vi "Create Tables.vi"() -> ()   [LabVIEW 2014, in "DB-Configuration.lvlib"]
doc: "This is a utilitiy VI to create necessary configuration tables in Oracle."
uses:
  DB-Configuration.lvlib
  <vilib>/addons/database/Auxilliary.llb/DB Tools Column Info.ctl
  <vilib>/addons/database/Auxilliary.llb/DB Tools DataTypes.ctl
  <vilib>/addons/database/Auxilliary.llb/DB Tools Transaction.ctl
  <vilib>/addons/database/Connection.llb/DB Tools Open Connec (String).vi
  <vilib>/addons/database/Connection.llb/Conn Transaction.vi
  <vilib>/addons/database/Connection.llb/Conn Execute.vi
  <vilib>/addons/database/Recordset.llb/Rec Destroy - Connection.vi
  <vilib>/addons/database/NI_Database_API.lvlib
panel:
  out "OK?":bool
  # "Create configuration tables in Oracle\nand insert demo data."
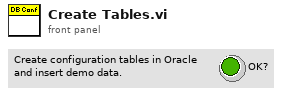
[diagram p1: front panel]
types:
  T1 = typedef "NI_Database_API.lvlib/DB Tools Transaction.ctl" = enum16{"begin", "commit", "rollback"}
  T2 = typedef "NI_Database_API.lvlib/DB Tools Column Info.ctl" = cluster{"column name":string, "data type":T3, "size":i32, "allow null?":bool}
  T3 = typedef "NI_Database_API.lvlib/DB Tools DataTypes.ctl" = enum16{"String", "Long (I32)", "Single (SGL)", "Double (DBL)", "Date/Time", "Binary"}
  T4 = typedef "NI_Database_API.lvlib/Conn ObjectReference.ctl" = refnum<k1>
  T5 = typedef "NI_Database_API.lvlib/Rec ObjectReference.ctl" = refnum<k1>
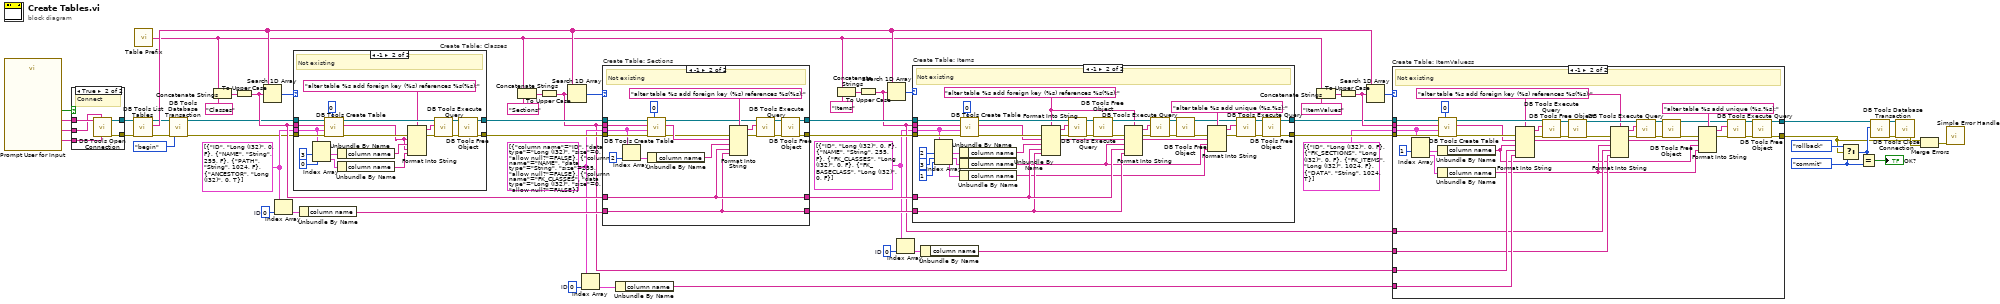
[diagram p0: block diagram]
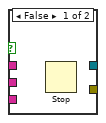
[diagram p6: hidden frame]
diagram:
  w5 = DB_Tools_Transaction."commit" ("operation (begin)")
  w20 = 0  # ID
  w24 = 0  # ID
  w33 = 0  # ID
  w22 = T2[] [{"column name"="ID", "data type"=enum."Long (I32)", "size"=0, "allow null?"=FALSE}, {"column name"="NAME", "data type"=enum."String", "size"=255, "allow null?"=FALSE}, {"column name"="FK_CLASSES", "data type"=enum."Long (I32)", "size"=0, "allow null?"=FALSE}, {"column name"="FK_BASECLASS", "data type"=enum."Long (I32)", "size"=0, "allow null?"=FALSE}] ("column information")
  w23 = T2[] [{"column name"="ID", "data type"=enum."Long (I32)", "size"=0, "allow null?"=FALSE}, {"column name"="NAME", "data type"=enum."String", "size"=255, "allow null?"=FALSE}, {"column name"="FK_CLASSES", "data type"=enum."Long (I32)", "size"=0, "allow null?"=FALSE}] ("column information")
  w31 = T2[] [{"column name"="ID", "data type"=enum."Long (I32)", "size"=0, "allow null?"=FALSE}, {"column name"="NAME", "data type"=enum."String", "size"=255, "allow null?"=FALSE}, {"column name"="PATH", "data type"=enum."String", "size"=1024, "allow null?"=FALSE}, {"column name"="ANCESTOR", "data type"=enum."Long (I32)", "size"=0, "allow null?"=TRUE}] ("column information")
  n1 = call "Prompt User for Input"() -> ("Password"=w58:string, "User Name"=w59:string, "ODBC Name"=w60:string, "OK"=w57:bool)  [unwired: 15 in, 1 out]
  n2 = case shown="True" w57 {
    tunnel: w60 -> [_ w65]
    tunnel: w59 -> [_ w64]
    tunnel: w58 -> [_ w63]
    tunnel: [_ w62] -> w56
    tunnel: [_ w61] -> w55
    frame False {
      n3 = Stop() -> ()  [unwired: 1 in]
    }
    frame True {
      # "Connect"
      n4 = call-poly <vilib>:"DB Tools Open Connection.vi"("password"=w63, "userID"=w64, "connection information"=w65) -> ("error out"=w61:errorcluster, "connection reference"=w62:T4)  [unwired: 5 in]
    }
  }
  n5 = call <vilib>:"DB Tools List Tables.vi"("error in (no error)"=w55, "connection reference"=w56) -> ("error out"=w13:errorcluster, "tables"=w37:string[], "connection reference out"=w15:T4)  [unwired: 3 in]
  n6 = call "Table Prefix.vi"() -> ("DB Table Prefix"=w16:string)
  n7 = call-poly <vilib>:"DB Tools Database Transaction.vi"("error in (no error)"=w13, "operation (begin)"=DB_Tools_Transaction."begin", "connection reference"=w15) -> ("error out"=w12:errorcluster, "connection reference out"=w14:T4)  [unwired: 3 in]
  n8 = Concatenate Strings(w16, "Classes" ("table")) -> (w52:string)
  n9 = To Upper Case(1:w52) -> (0:w34:string)
  n10 = Search 1D Array(1D array=w37, element=w34) -> (index of element=w53:i32)  [unwired: 1 in]
  n11 = Index Array(array=w31, index=w33) -> (element=w32:T2)
  n12 = case "Create Table: Classes" shown="-1" w53 {
    tunnel: w14 -> [w67 w87]
    tunnel: w12 -> [w66 w86]
    tunnel: w34 -> [_ w71]
    tunnel: [w67 w78] -> w48
    tunnel: [w66 w77] -> w47
    tunnel: w31 -> [_ w74]
    frame 0, Default {
    }
    frame -1 {
      # "Not existing"
      n13 = Index Array(array=w74, index #1=3 ("index"), index #2=0 ("index")) -> (element #1=w76:T2, element #2=w69:T2)
      n14 = call <vilib>:"DB Tools Create Table.vi"("primary key (-1)"=0, "error in (no error)"=w86, "column information"=w74, "table"=w71, "connection reference"=w87) -> ("error out"=w81:errorcluster, "connection reference out"=w80:T4)  [unwired: 3 in]
      n15 = Unbundle By Name(w76) -> ("column name"=w72:string)
      n16 = Unbundle By Name(w69) -> ("column name"=w68:string)
      n17 = Format Into String(format string="alter table %s add foreign key (%s) references %s(%s);" ("SQL query"), error in=w81, w71, w72, w71, w68) -> (resulting string=w83:string, error out=w84:errorcluster)  [unwired: 1 in]
      n18 = call-poly <vilib>:"DB Tools Execute Query.vi"("error in (no error)"=w84, "SQL query"=w83, "connection reference"=w80) -> ("error out"=w82:errorcluster, "recordset reference"=w79:T5)  [unwired: 5 in]
      n19 = call-poly <vilib>:"DB Tools Free Object.vi"("error in (no error)"=w82, "recordset reference"=w79) -> ("error out"=w77:errorcluster, "connection reference"=w78:T4)  [unwired: 8 in]
    }
  }
  n20 = Unbundle By Name(w32) -> ("column name"=w30:string)
  n21 = Concatenate Strings(w16, "Sections" ("table")) -> (w51:string)
  n22 = To Upper Case(1:w51) -> (0:w19:string)
  n23 = Search 1D Array(1D array=w37, element=w19) -> (index of element=w50:i32)  [unwired: 1 in]
  n24 = Index Array(array=w23, index=w24) -> (element=w25:T2)
  n25 = case "Create Table: Sections" shown="-1" w50 {
    tunnel: w48 -> [w91 w110]
    tunnel: w47 -> [w90 w109]
    tunnel: w19 -> [_ w105]
    tunnel: [w91 w98] -> w36
    tunnel: [w90 w101] -> w35
    tunnel: w23 -> [_ w94]
    tunnel: w30 -> [w88 w92]
    tunnel: w34 -> [w89 w93]
    tunnel: [w89 w93] -> w29
    tunnel: [w88 w92] -> w28
    frame 0, Default {
    }
    frame -1 {
      # "Not existing"
      n26 = Index Array(array=w94, index=2) -> (element=w96:T2)
      n27 = call <vilib>:"DB Tools Create Table.vi"("primary key (-1)"=0, "error in (no error)"=w109, "column information"=w94, "table"=w105, "connection reference"=w110) -> ("error out"=w100:errorcluster, "connection reference out"=w99:T4)  [unwired: 3 in]
      n28 = Unbundle By Name(w96) -> ("column name"=w95:string)
      n29 = Format Into String(format string="alter table %s add foreign key (%s) references %s(%s);" ("SQL query"), error in=w100, w105, w95, w93, w92) -> (resulting string=w103:string, error out=w102:errorcluster)  [unwired: 1 in]
      n30 = call-poly <vilib>:"DB Tools Execute Query.vi"("error in (no error)"=w102, "SQL query"=w103, "connection reference"=w99) -> ("error out"=w106:errorcluster, "recordset reference"=w107:T5)  [unwired: 5 in]
      n31 = call-poly <vilib>:"DB Tools Free Object.vi"("error in (no error)"=w106, "recordset reference"=w107) -> ("error out"=w101:errorcluster, "connection reference"=w98:T4)  [unwired: 8 in]
    }
  }
  n32 = Unbundle By Name(w25) -> ("column name"=w18:string)
  n33 = Concatenate Strings(w16, "Items" ("table")) -> (w44:string)
  n34 = To Upper Case(1:w44) -> (0:w26:string)
  n35 = Search 1D Array(1D array=w37, element=w26) -> (index of element=w45:i32)  [unwired: 1 in]
  n36 = Index Array(array=w22, index=w20) -> (element=w21:T2)
  n37 = case "Create Table: Items" shown="-1" w45 {
    tunnel: w36 -> [w112 w150]
    tunnel: w35 -> [w111 w142]
    tunnel: w26 -> [_ w123]
    tunnel: [w112 w135] -> w39
    tunnel: [w111 w136] -> w38
    tunnel: w22 -> [_ w141]
    tunnel: w29 -> [_ w120]
    tunnel: w28 -> [_ w119]
    frame 0, Default {
    }
    frame -1 {
      w125 = "alter table %s add foreign key (%s) references %s(%s);" ("SQL query")
      # "Not existing"
      n38 = Index Array(array=w141, index #1=2 ("index"), index #2=3 ("index"), index #3=1 ("index")) -> (element #1=w148:T2, element #2=w132:T2, element #3=w121:T2)
      n39 = Unbundle By Name(w148) -> ("column name"=w131:string)
      n40 = Unbundle By Name(w132) -> ("column name"=w114:string)
      n41 = Unbundle By Name(w121) -> ("column name"=w113:string)
      n42 = call <vilib>:"DB Tools Create Table.vi"("primary key (-1)"=0, "error in (no error)"=w142, "column information"=w141, "table"=w123, "connection reference"=w150) -> ("error out"=w139:errorcluster, "connection reference out"=w140:T4)  [unwired: 3 in]
      n43 = Format Into String(format string=w125, error in=w139, w123, w131, w120, w119) -> (resulting string=w145:string, error out=w146:errorcluster)  [unwired: 1 in]
      n44 = call-poly <vilib>:"DB Tools Execute Query.vi"("error in (no error)"=w146, "SQL query"=w145, "connection reference"=w140) -> ("error out"=w144:errorcluster, "recordset reference"=w143:T5)  [unwired: 5 in]
      n45 = call-poly <vilib>:"DB Tools Free Object.vi"("error in (no error)"=w144, "recordset reference"=w143) -> ("error out"=w124:errorcluster, "connection reference"=w126:T4)  [unwired: 8 in]
      n46 = Format Into String(format string=w125, error in=w124, w123, w114, w120, w119) -> (resulting string=w127:string, error out=w115:errorcluster)  [unwired: 1 in]
      n47 = call-poly <vilib>:"DB Tools Execute Query.vi"("error in (no error)"=w115, "SQL query"=w127, "connection reference"=w126) -> ("error out"=w116:errorcluster, "recordset reference"=w128:T5)  [unwired: 5 in]
      n48 = call-poly <vilib>:"DB Tools Free Object.vi"("error in (no error)"=w116, "recordset reference"=w128) -> ("error out"=w117:errorcluster, "connection reference"=w118:T4)  [unwired: 8 in]
      n49 = Format Into String(format string="alter table %s add unique (%s,%s);" ("SQL query"), error in=w117, w123, w114, w113) -> (resulting string=w130:string, error out=w134:errorcluster)  [unwired: 1 in]
      n50 = call-poly <vilib>:"DB Tools Execute Query.vi"("error in (no error)"=w134, "SQL query"=w130, "connection reference"=w118) -> ("error out"=w137:errorcluster, "recordset reference"=w138:T5)  [unwired: 5 in]
      n51 = call-poly <vilib>:"DB Tools Free Object.vi"("error in (no error)"=w137, "recordset reference"=w138) -> ("error out"=w136:errorcluster, "connection reference"=w135:T4)  [unwired: 8 in]
    }
  }
  n52 = Unbundle By Name(w21) -> ("column name"=w17:string)
  n53 = Concatenate Strings(w16, "ItemValues" ("table")) -> (w42:string)
  n54 = To Upper Case(1:w42) -> (0:w43:string)
  n55 = Search 1D Array(1D array=w37, element=w43) -> (index of element=w41:i32)  [unwired: 1 in]
  n56 = case "Create Table: ItemValuess" shown="-1" w41 {
    tunnel: w39 -> [w152 w188]
    tunnel: w38 -> [w151 w187]
    tunnel: w43 -> [_ w155]
    tunnel: [w152 w157] -> w2
    tunnel: [w151 w156] -> w1
    tunnel: T2[] [{"column name"="ID", "data type"=enum."Long (I32)", "size"=0, "allow null?"=FALSE}, {"column name"="FK_SECTIONS", "data type"=enum."Long (I32)", "size"=0, "allow null?"=FALSE}, {"column name"="FK_ITEMS", "data type"=enum."Long (I32)", "size"=1024, "allow null?"=FALSE}, {"column name"="DATA", "data type"=enum."String", "size"=1024, "allow null?"=TRUE}] ("column information") -> [_ w183]
    tunnel: w26 -> [_ w167]
    tunnel: w19 -> [_ w176]
    tunnel: w18 -> [_ w175]
    tunnel: w17 -> [_ w166]
    frame 0, Default {
    }
    frame -1 {
      w168 = "alter table %s add foreign key (%s) references %s(%s);" ("SQL query")
      # "Not existing"
      n57 = Index Array(array=w183, index #1=1 ("index")) -> (element #1=w184:T2, element #2=w182:T2)  [unwired: 1 in]
      n58 = Unbundle By Name(w184) -> ("column name"=w154:string)
      n59 = Unbundle By Name(w182) -> ("column name"=w153:string)
      n60 = call <vilib>:"DB Tools Create Table.vi"("primary key (-1)"=0, "error in (no error)"=w187, "column information"=w183, "table"=w155, "connection reference"=w188) -> ("error out"=w165:errorcluster, "connection reference out"=w177:T4)  [unwired: 3 in]
      n61 = Format Into String(format string=w168, error in=w165, w155, w154, w176, w175) -> (resulting string=w179:string, error out=w178:errorcluster)  [unwired: 1 in]
      n62 = call-poly <vilib>:"DB Tools Execute Query.vi"("error in (no error)"=w178, "SQL query"=w179, "connection reference"=w177) -> ("error out"=w180:errorcluster, "recordset reference"=w181:T5)  [unwired: 5 in]
      n63 = call-poly <vilib>:"DB Tools Free Object.vi"("error in (no error)"=w180, "recordset reference"=w181) -> ("error out"=w169:errorcluster, "connection reference"=w170:T4)  [unwired: 8 in]
      n64 = Format Into String(format string=w168, error in=w169, w155, w153, w167, w166) -> (resulting string=w173:string, error out=w174:errorcluster)  [unwired: 1 in]
      n65 = call-poly <vilib>:"DB Tools Execute Query.vi"("error in (no error)"=w174, "SQL query"=w173, "connection reference"=w170) -> ("error out"=w172:errorcluster, "recordset reference"=w171:T5)  [unwired: 5 in]
      n66 = call-poly <vilib>:"DB Tools Free Object.vi"("error in (no error)"=w172, "recordset reference"=w171) -> ("error out"=w158:errorcluster, "connection reference"=w159:T4)  [unwired: 8 in]
      n67 = Format Into String(format string="alter table %s add unique (%s,%s);" ("SQL query"), error in=w158, w155, w154, w153) -> (resulting string=w163:string, error out=w162:errorcluster)  [unwired: 1 in]
      n68 = call-poly <vilib>:"DB Tools Execute Query.vi"("error in (no error)"=w162, "SQL query"=w163, "connection reference"=w159) -> ("error out"=w161:errorcluster, "recordset reference"=w160:T5)  [unwired: 5 in]
      n69 = call-poly <vilib>:"DB Tools Free Object.vi"("error in (no error)"=w161, "recordset reference"=w160) -> ("error out"=w156:errorcluster, "connection reference"=w157:T4)  [unwired: 8 in]
    }
  }
  n70 = Select(t=DB_Tools_Transaction."rollback" ("operation (begin)"), s=w1, f=w5) -> (s? t:f=w6:T1)
  n71 = Equal?(x=w6, y=w5) -> (x = y?=→"OK?":bool)
  n72 = call-poly <vilib>:"DB Tools Database Transaction.vi"("operation (begin)"=w6, "connection reference"=w2) -> ("error out"=w9:errorcluster, "connection reference out"=w10:T4)  [unwired: 4 in]
  n73 = call <vilib>:"DB Tools Close Connection.vi"("error in (no error)"=w9, "connection reference"=w10) -> ("error out"=w3:errorcluster)  [unwired: 5 in]
  n74 = Merge Errors(w1, w3) -> (w7:errorcluster)
  n75 = call <vilib>:"Simple Error Handler.vi"("error in (no error)"=w7) -> ()  [unwired: 4 in, 5 out]
